vi "Untitled 1 (SubVI).vi"(6 "Sampling freq.":i32, 9 "Carrier Frequency":i32, 10 "number of bits":dbl, 11 "Number of Cycles":i32) -> (1 "output":dbl[](graph), 2 "Modulating Square Chart":i8(graph), 3 "Modulating Square":i8[](graph), 4 "Carrier":dbl[](graph), 5 "Output Chart":dbl(graph))   [LabVIEW 2015]
panel:
  in  "Numeric":i32
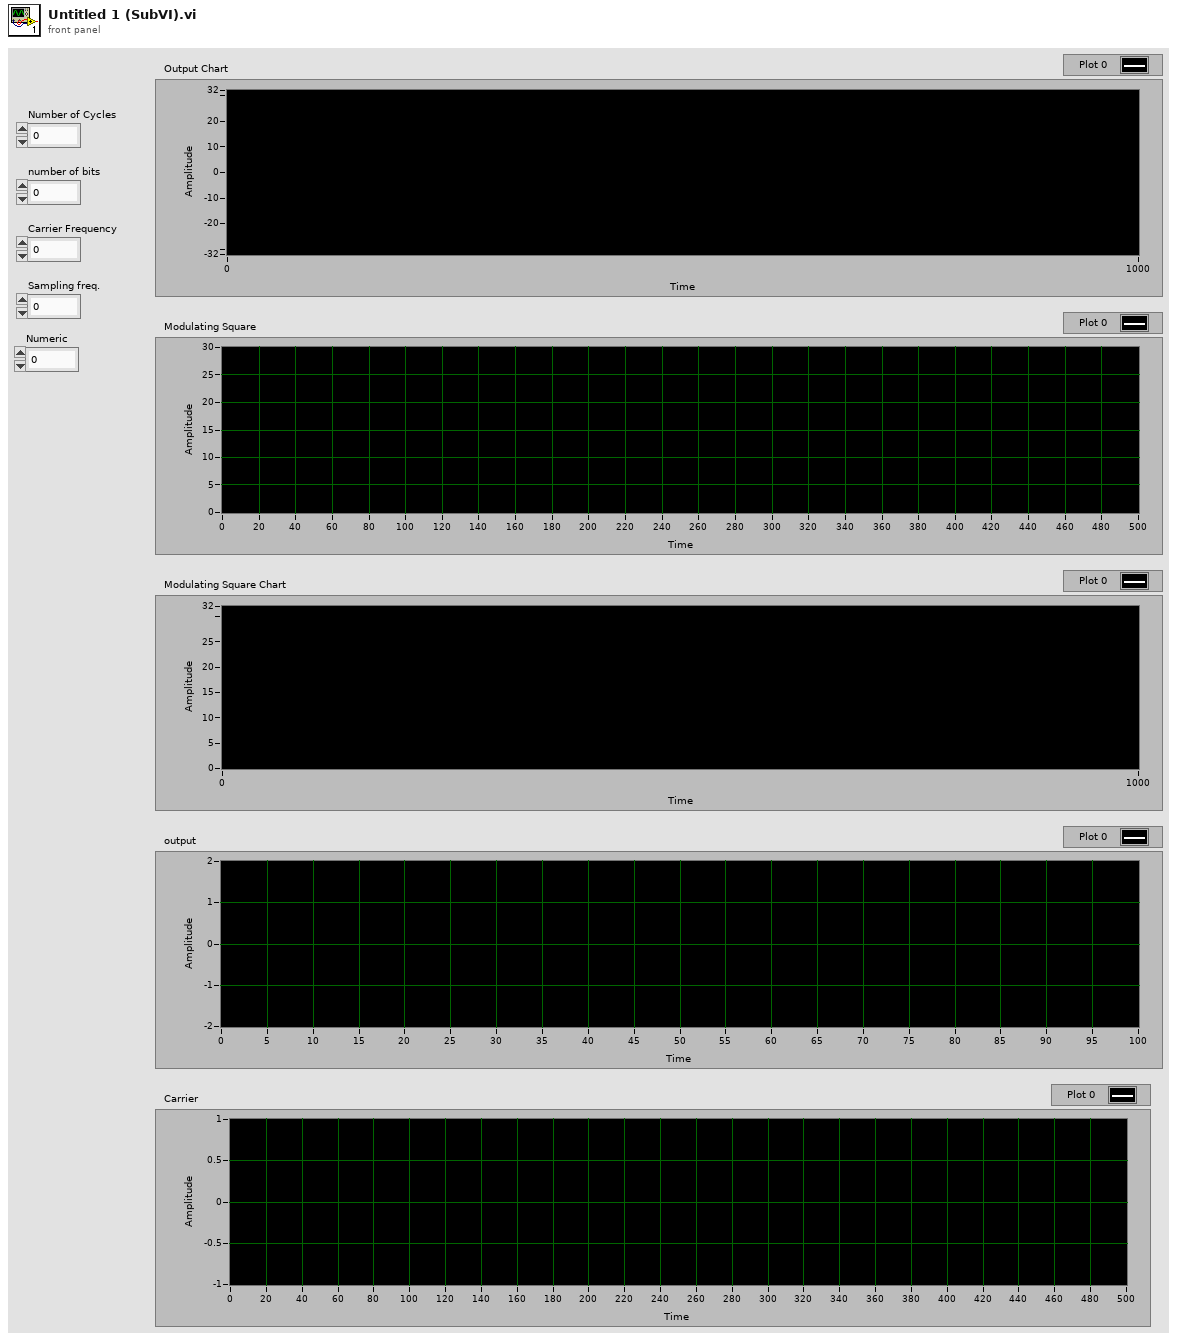
[diagram p1: front panel]
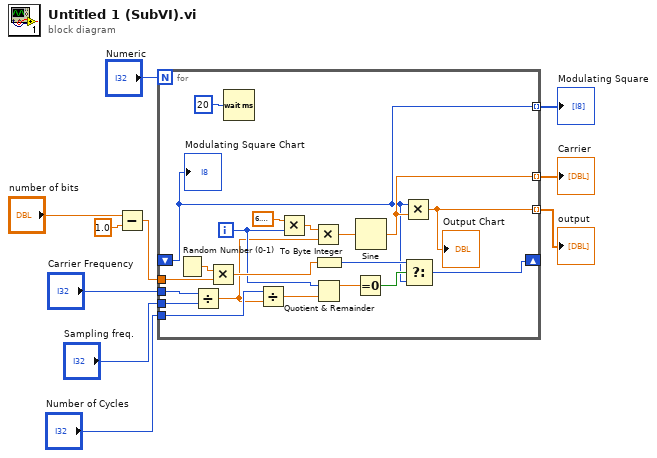
[diagram p0: block diagram]
diagram:
  n1 = Subtract(x="number of bits", y=1.0) -> (x-y=w2:dbl)
  n2 = for {
    N: "Numeric" -> [_]
    tunnel: "Sampling freq." -> [w30]
    tunnel: "Carrier Frequency" -> [w18]
    tunnel: [w13] -> w7 mode=indexing
    tunnel: [w28] -> w8 mode=indexing
    tunnel: w2 -> [w26]
    shift-right: [w20] -> _
    shift-left: _ -> [w11]
    tunnel: "Number of Cycles" -> [w16]
    tunnel: [w11] -> w10 mode=indexing
    i -> [w17]
    n3 = Random Number (0-1)() -> (number: 0 to 1=w27:dbl)
    n4 = Divide(x=w18, y=w30) -> (x/y=w15:dbl)
    n5 = Multiply(x=w27, y=w26) -> (x*y=w25:dbl)
    n6 = Wait (ms)(milliseconds to wait=u32 20) -> ()  [unwired: 1 out]
    n7 = Divide(x=w16, y=w15) -> (x/y=w14:dbl)
    n8 = Multiply(x=6.283185307179586, y=w17) -> (x*y=w24:dbl)
    n9 = Multiply(x=w24, y=w15) -> (x*y=w29:dbl)
    n10 = To Byte Integer(number=w25) -> (8bit integer=w21:i8)
    n11 = Quotient & Remainder(x=w17, y=w14) -> (x-y*floor(x/y)=w23:dbl)  [unwired: 1 out]
    n12 = Equal To 0?(x=w23) -> (x = 0?=w22:bool)
    n13 = Sine(x=w29) -> (sin(x)=w28:dbl)
    n14 = Multiply(x=w11, y=w28) -> (x*y=w13:dbl)
    "Output Chart" <- w13
    n15 = Select(t=w21, s=w22, f=w11) -> (s? t:f=w20:i8)
    "Modulating Square Chart" <- w11
  }
  "output" <- w7
  "Carrier" <- w8
  "Modulating Square" <- w10
